vi "Temperature Warnings.vi"(8 "error in (no error)":errorcluster, 9 "Min Temperature":dbl, 10 "Max Temperature":dbl, 11 "Current Temperature":dbl) -> (0 "error out":errorcluster, 2 "Warning Text":string="No Warning", 3 "Warning?":bool)   [LabVIEW 2015]
doc: "This VI is used to determine the string to output to the weather station based on the current temperature and limit settings.\n\nInputs: Current Temperature (DBL), Minimum Temperature (DBL), and Maximum Temperature (DBL).\nOutputs: Warning Text (string) and Warning? (Boolean)."
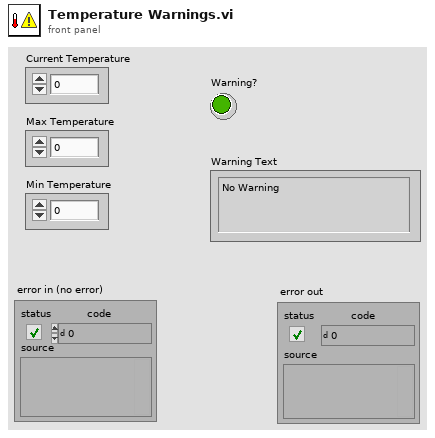
[diagram p1: front panel]
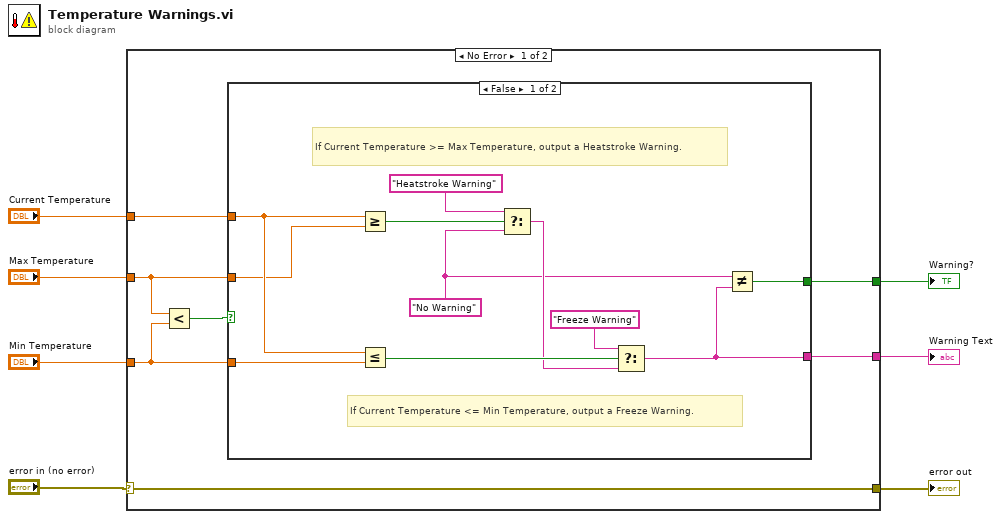
[diagram p0: block diagram]
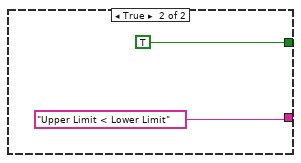
[diagram p2: hidden frame]
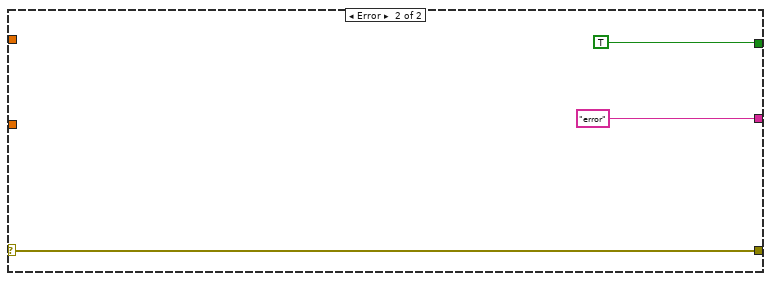
[diagram p3: hidden frame]
diagram:
  n1 = case shown="No Error" "error in (no error)" {
    selector: "error in (no error)" -> [w8 w28]
    tunnel: "Current Temperature" -> [w14 _]
    tunnel: [w13 TRUE] -> w6
    tunnel: [w12 "error"] -> w5
    tunnel: "Max Temperature" -> [w11 _]
    tunnel: "Min Temperature" -> [w10 _]
    tunnel: [w8 w28] -> w1
    frame No Error {
      n2 = Less?(x=w11, y=w10) -> (x < y?=w9:bool)
      n3 = case shown="False" w9 {
        tunnel: w14 -> [w25 _]
        tunnel: w10 -> [w24 _]
        tunnel: w11 -> [w23 _]
        tunnel: [w22 TRUE] -> w13
        tunnel: [w21 "Upper Limit < Lower Limit"] -> w12
        frame False {
          w15 = "No Warning" ("f")
          # "If Current Temperature >= Max Temperature, output a Heatstroke Warning."
          # "If Current Temperature <= Min Temperature, output a Freeze Warning."
          n4 = Greater Or Equal?(x=w25, y=w23) -> (x >= y?=w20:bool)
          n5 = Less Or Equal?(x=w25, y=w24) -> (x <= y?=w17:bool)
          n6 = Select(t="Heatstroke Warning", s=w20, f=w15) -> (s? t:f=w16:string)
          n7 = Select(t="Freeze Warning", s=w17, f=w16) -> (s? t:f=w21:string)
          n8 = Not Equal?(x=w15, y=w21) -> (x != y?=w22:bool)
        }
        frame True {
        }
      }
    }
    frame Error {
    }
  }
  "Warning?" <- w6
  "Warning Text" <- w5
  "error out" <- w1
